vi "SettingsEngine.vi"(7 "Enum":T1, 8 "error in":errorcluster, 9 "Dir for Settings File":path, 10 "New Setting Value":string, 11 "Setting Name":string) -> (0 "error out":errorcluster, 2 "Setting Value":string)   [LabVIEW 8.6]
uses:
  SettingsEngineEnum.ctl
panel:
  out "array":string[][](array[string])
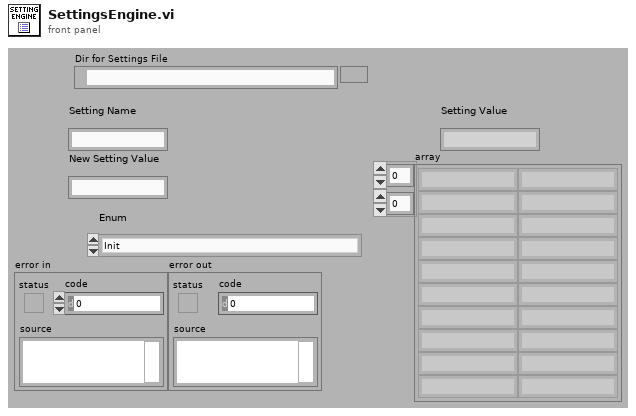
[diagram p1: front panel]
types:
  T1 = typedef "SettingsEngineEnum.ctl" = enum16{"Init", "Load Settings from File", "Get Setting", "Set/Create Setting", "Save Settings to File"}
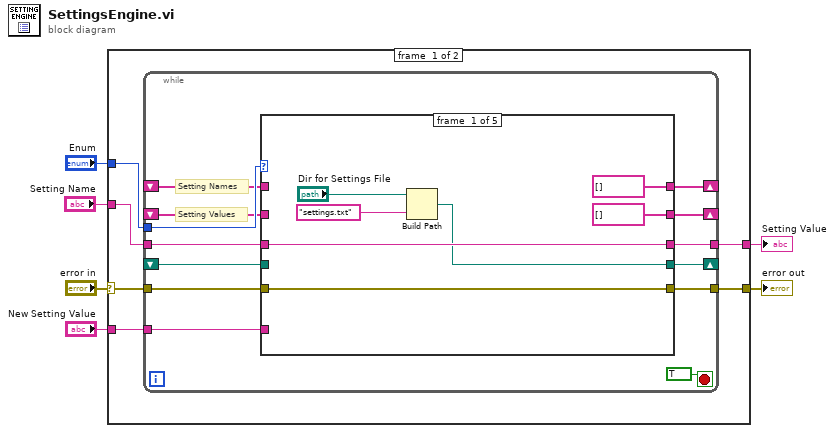
[diagram p0: block diagram]
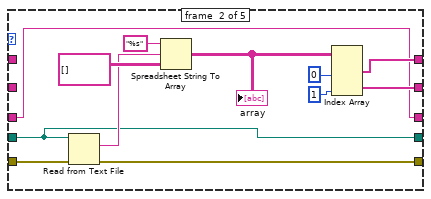
[diagram p2: hidden frame]
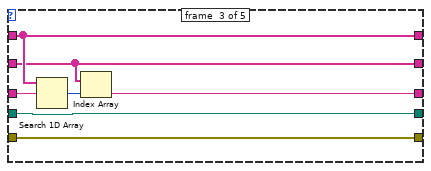
[diagram p3: hidden frame]
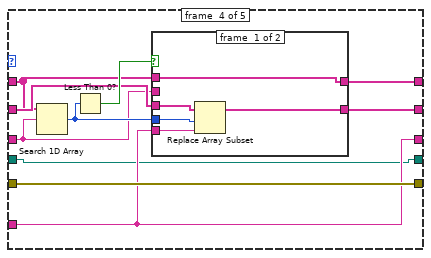
[diagram p4: hidden frame]
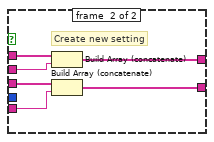
[diagram p5: hidden frame]
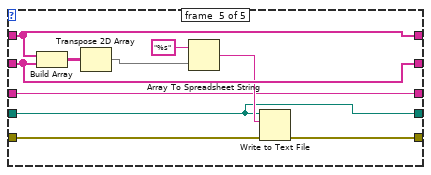
[diagram p6: hidden frame]
diagram:
  n1 = case shown="No Error" "error in" {
    selector: "error in" -> [w11 w84]
    tunnel: "Enum" -> [w12 _]
    tunnel: [w10 w84] -> w4
    tunnel: "Setting Name" -> [w9 w83]
    tunnel: [w8 w83] -> w2
    tunnel: "New Setting Value" -> [w7 _]
    frame #0 {
      n2 = while {
        tunnel: w12 -> [w24]
        shift-right: [w23] -> _
        shift-left: _ -> [w22]
        shift-right: [w21] -> _
        shift-left: _ -> [w20]
        tunnel: w11 -> [w19]
        tunnel: [w18] -> w10
        tunnel: w9 -> [w16]
        tunnel: [w15] -> w8
        tunnel: w7 -> [w14]
        shift-right: [w13] -> _
        shift-left: _ -> [w17]
        stop <- TRUE ("stop") stop-if-true
        # "Setting Values"
        # "Setting Names"
        n3 = case shown="\"Init\", Default" w24 {
          tunnel: [string[] [] w36 w50 w55 w82] -> w23
          tunnel: w22 -> [_ _ w50 w54 w82]
          tunnel: [string[] [] w35 w48 w56 w81] -> w21
          tunnel: w20 -> [_ _ w48 w59 w81]
          tunnel: w19 -> [w30 w44 w51 w61 w76]
          tunnel: [w30 w43 w51 w61 w75] -> w18
          tunnel: w17 -> [_ w33 w45 w52 w73]
          tunnel: w16 -> [w29 w34 w49 w53 w74]
          tunnel: [w29 w34 w46 w58 w74] -> w15
          tunnel: w14 -> [_ _ _ w58 _]
          tunnel: [w26 w33 w45 w52 w73] -> w13
          frame #0 {
            n4 = Build Path(base path="Dir for Settings File", name or relative path="settings.txt") -> (appended path=w26:path)
          }
          frame #1 {
            n5 = Read from Text File(file (use dialog)=w33, error in=w44) -> (text=w41:string, error out=w43:errorcluster)  [unwired: 2 in, 2 out]
            n6 = Spreadsheet String To Array(format string="%s", spreadsheet string=w41, array type (2D Dbl)=string[][] []) -> (array=w39:string[][])  [unwired: 1 in]
            "array" <- w39
            n7 = Index Array(array=w39, index (col) #1=0 ("disabled index (col)"), index (col) #2=1 ("index (col)")) -> (element #1=w36:string[], element #2=w35:string[])  [unwired: 2 in]
          }
          frame #2 {
            n8 = Search 1D Array(1D array=w50, element=w49) -> (index of element=w47:i32)  [unwired: 1 in]
            n9 = Index Array(array=w48, index=w47) -> (element=w46:string)
          }
          frame #3 {
            n10 = Search 1D Array(1D array=w54, element=w53) -> (index of element=w57:i32)  [unwired: 1 in]
            n11 = Less Than 0?(x=w57) -> (x < 0?=w60:bool)
            n12 = case shown="True" w60 {
              tunnel: w59 -> [w66 w70]
              tunnel: w58 -> [w65 w67]
              tunnel: w57 -> [w64 _]
              tunnel: [w63 w69] -> w56
              tunnel: [w62 w71] -> w55
              tunnel: w54 -> [w62 w72]
              tunnel: w53 -> [_ w68]
              frame #0 {
                n13 = Replace Array Subset(array=w66, new element=w65, index=w64) -> (w63:string[])
              }
              frame #1 {
                # "Create new setting"
                n14 = Build Array (concatenate)(w72, w68) -> (w71:string[])
                n15 = Build Array (concatenate)(w70, w67) -> (w69:string[])
              }
            }
          }
          frame #4 {
            n16 = Build Array(w82, w81) -> (w79:string[][])
            n17 = Transpose 2D Array(2D array=w79) -> (transposed array=w78:string[][])
            n18 = Array To Spreadsheet String(array=w78, 3:"%s" ("format string")) -> (spreadsheet string=w77:string)  [unwired: 1 in]
            n19 = Write to Text File(file (use dialog)=w73, text=w77, error in=w76) -> (error out=w75:errorcluster)  [unwired: 1 in, 2 out]
          }
        }
      }
    }
    frame #1 {
    }
  }
  "error out" <- w4
  "Setting Value" <- w2
